vi "Write Angel (rad).vi"(10 "Angel (rad)":dbl, 11 "ValveModbus in":refnum<class "NeedleValve.lvclass">) -> (3 "ValveModbus out":refnum<class "NeedleValve.lvclass">)   [LabVIEW 2019, in "NeedleValve.lvclass"]
uses:
  NeedleValve.lvclass
  NeedleValve.lvclass/NeedleValve.ctl
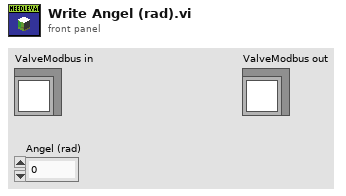
[diagram p1: front panel]
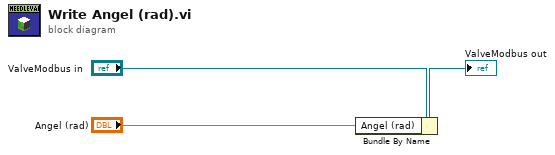
[diagram p0: block diagram]
diagram:
  n1 = Bundle By Name(cluster="ValveModbus in", "Angel (rad)"="Angel (rad)") -> (→"ValveModbus out":refnum<class "NeedleValve.lvclass">)
